vi "dfd_Generate Quantized Coef Report Header.vi"(8 "error in (no error)":errorcluster) -> (0 "error out":errorcluster, 2 "coef report header":string)   [LabVIEW 2017, in "NI_DigFilter_FXP.lvlib"]
uses:
  <vilib>/addons/Digital Filter Design/NI_DigFilter_FXP.lvlib
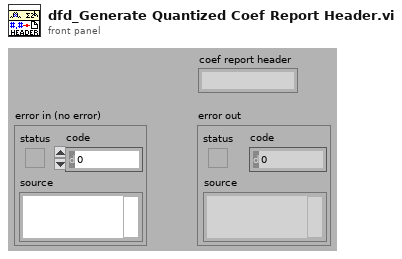
[diagram p1: front panel]
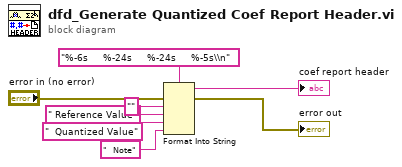
[diagram p0: block diagram]
diagram:
  n1 = Format Into String(format string="%-6s     %-24s     %-24s     %-5s\\n", error in="error in (no error)", "" ("input 1"), " Reference Value" ("input 2"), "  Quantized Value" ("input 3"), "  Note" ("input 4")) -> (resulting string=→"coef report header":string, error out=→"error out":errorcluster)  [unwired: 1 in]
